vi "Jump_Globals.vi"() -> ()   [LabVIEW 2021]
panel:
  in  "Jump 6":dbl[](array[numeric])
  in  "Jump 5":dbl[](array[numeric])
  in  "Jump 4":dbl[](array[numeric])
  in  "Jump 3":dbl[](array[numeric])
  in  "Jump 2":dbl[](array[numeric])
  in  "Jump 1":dbl[](array[numeric])
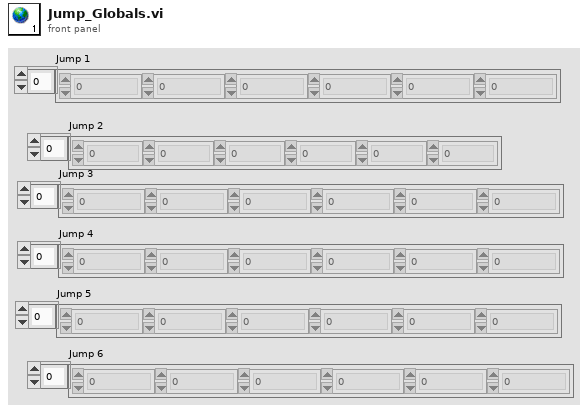
[diagram p1: front panel]
diagram:
